vi "Main.vi"(8 "error in (no error)":errorcluster) -> (0 "error out":errorcluster)   [LabVIEW 2020]
doc: "ATM machine CLA Exam !\nHappy new year from France !!!!!!! :)"
uses:
  FGV/Controls/FGV_State.ctl
panel:
  # "This VI is the launcher for ATM machine exam.\nIt manage all the program by initializing communications element, lauching modules and starting automatoically all UI"
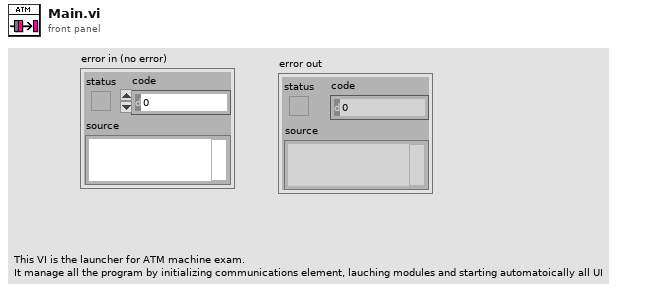
[diagram p1: front panel]
types:
  T1 = typedef "FGV_State.ctl" = enum16{"1 - OpenDatabase", "2 - Initialize Events", "3 - Initialize QMH", "4 - Close QMH", "5 - Close Events", "Read FGV", "Save Database", "Def"}
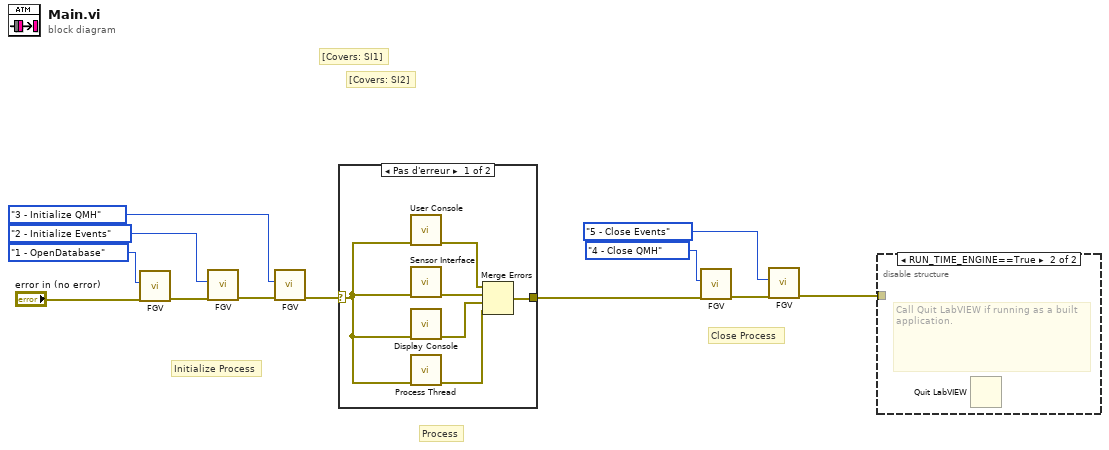
[diagram p0: block diagram]
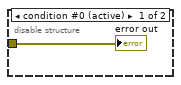
[diagram p3: hidden frame]
diagram:
  # "[Covers: SI2]"
  # "[Covers: SI1]"
  # "Process"
  # "Close Process"
  # "Initialize Process"
  n1 = call "FGV.vi"("error in (no error)"="error in (no error)", "FGV_State"=FGV_State."1 - OpenDatabase") -> ("error out"=w10:errorcluster)  [unwired: 8 in, 1 out]
  n2 = call "FGV.vi"("error in (no error)"=w10, "FGV_State"=FGV_State."2 - Initialize Events") -> ("error out"=w9:errorcluster)  [unwired: 8 in, 1 out]
  n3 = call "FGV.vi"("error in (no error)"=w9, "FGV_State"=FGV_State."3 - Initialize QMH") -> ("error out"=w7:errorcluster)  [unwired: 8 in, 1 out]
  n4 = case shown="Pas d'erreur" w7 {
    selector: w7 -> [w14 w19]
    tunnel: [w15 w19] -> w3
    frame No Error {
      n5 = call "User Console.vi"("error in"=w14) -> ("error out"=w18:errorcluster)  [unwired: 10 in]
      n6 = call "Sensor Interface.vi"("error in (no error)"=w14) -> ("error out"=w17:errorcluster)  [unwired: 10 in]
      n7 = call "Display Console.vi"("error in (no error)"=w14) -> ("error out"=w16:errorcluster)  [unwired: 10 in]
      n8 = call "Process Thread.vi"("error in (no error)"=w14) -> ("error out"=w13:errorcluster)  [unwired: 10 in]
      n9 = Merge Errors(w18, w17, w16, w13) -> (w15:errorcluster)
    }
    frame Error {
    }
  }
  n10 = call "FGV.vi"("error in (no error)"=w3, "FGV_State"=FGV_State."4 - Close QMH") -> ("error out"=w6:errorcluster)  [unwired: 8 in, 1 out]
  n11 = call "FGV.vi"("error in (no error)"=w6, "FGV_State"=FGV_State."5 - Close Events") -> ("error out"=w1:errorcluster)  [unwired: 8 in, 1 out]
  n12 = disable-structure shown="RUN_TIME_ENGINE==True" {
    disable-tunnel: w1 -> [w20 _]
    frame condition #0 (active) {
      "error out" <- w20
    }
    frame condition #1 {
      # "Call Quit LabVIEW if running as a built application."
      n13 = Quit LabVIEW() -> ()  [unwired: 1 in]
    }
  }
